vi "Configure PAS.vi"(8 "error in (no error)":errorcluster, 11 "Controller In":refnum<class "gController.lvclass">) -> ()   [LabVIEW 2017, in "Controller.lvlib" / "gController.lvclass"]
uses:
  gController.lvclass
  C:/Program Files (x86)/National Instruments/LabVIEW 2017/vi.lib/MSR Consulting, LLC/General Reuse/SuperActor/SuperActor.lvclass
  C:/Program Files (x86)/National Instruments/LabVIEW 2017/vi.lib/ActorFramework/Actor/Actor.lvclass
  Messages/Change Heater Ctl Params MSG/Change Heater Ctl Params.lvclass
  C:/Program Files (x86)/National Instruments/LabVIEW 2017/vi.lib/ActorFramework/Message/Message.lvclass
  Messages/Change Heater SP MSG/Change Heater SP MSG.lvclass
  Messages/Update PAS Enable Laser State/Update PAS Laser 0 Enable State MSG.lvclass
  G:/sw_repo/For Builds/Nicholas/Controller/Messages/Generic Boolean MSG/Generic Boolean Message.lvclass
  Messages/Enable PAS Laser 1 MSG/Update PAS Laser 1 Enable State MSG.lvclass
  PAS/Commands/Change Speaker State Cmd/Change Speaker State CMD.lvclass
  C:/Program Files (x86)/National Instruments/LabVIEW 2017/vi.lib/MSR Consulting, LLC/General Reuse/PAS/Commands/Change Speaker State CMD/Change Speaker State CMD.lvclass
  C:/Program Files (x86)/National Instruments/LabVIEW 2017/vi.lib/MSR Consulting, LLC/General Reuse/Command/Command.lvclass
  Messages/Forward Command/Forward Command MSG.lvclass
  <vilib>/MSR Consulting, LLC/General Reuse/Session APIs/File Access/Config Data/Config Data.lvclass
  <vilib>/MSR Consulting, LLC/General Reuse/PAS/Commands/Change Speaker State CMD/Change Speaker State CMD.lvclass/Change Speaker State CMD.ctl
  Messages/Forward Command/Forward Command MSG.lvclass/Forward Command MSG.ctl
  <vilib>/MSR Consulting, LLC/General Reuse/SuperActor/SuperActor.lvclass/SuperActor.ctl
  <vilib>/ActorFramework/Actor/Actor.lvclass/Actor.ctl
  <vilib>/ActorFramework/Message Enqueuer/Message Enqueuer.lvclass/Message Enqueuer.ctl
  <vilib>/MSR Consulting, LLC/General Reuse/Session APIs/File Access/Config Data/Config Data.lvclass/Config Data.ctl
  Messages/Change Heater Ctl Params MSG/Change Heater Ctl Params.lvclass/Change Heater Ctl Params.ctl
  Messages/Generic Boolean MSG/Generic Boolean Message.lvclass/Generic Boolean Message.ctl
  Messages/Change Heater SP MSG/Change Heater SP MSG.lvclass/Change Heater SP MSG.ctl
  <vilib>/MSR Consulting, LLC/General Reuse/SuperActor/Read Config Session.vi
  <vilib>/MSR Consulting, LLC/General Reuse/PAS/Commands/Change Speaker State CMD/Write cell.vi
  <vilib>/MSR Consulting, LLC/General Reuse/PAS/Commands/Change Speaker State CMD/Write state.vi
  Messages/Forward Command/Write CMD.vi
  Messages/Forward Command/Write id.vi
  <vilib>/MSR Consulting, LLC/General Reuse/Session APIs/File Access/Config Data/Accessors/Read Ref.vi
  Messages/Generic Boolean MSG/Write Bool.vi
  Messages/Change Heater SP MSG/Write id.vi
  Messages/Change Heater SP MSG/Write sp.vi
  Messages/Change Heater Ctl Params MSG/Write id.vi
  Messages/Change Heater Ctl Params MSG/Write ctl.vi
  <vilib>/ActorFramework/Message Enqueuer/Init from Existing Queue.vi
  <vilib>/MSR Consulting, LLC/General Reuse/Session APIs/File Access/Config Data/Read Array/Read DBL Array.vi
  <vilib>/MSR Consulting, LLC/General Reuse/Session APIs/File Access/Config Data/Read Array/Read Boolean Array.vi
  <vilib>/Utility/config.llb/Read Key (Double).vi
  <vilib>/ActorFramework/Message Priority Queue/Priority Enqueue.vi
  <vilib>/MSR Consulting, LLC/General Reuse/Session APIs/_Session Fwk/Session - Root.lvclass
  <vilib>/ActorFramework/Message Enqueuer/Message Enqueuer.lvclass
  <vilib>/Utility/config.llb/NI_LVConfig.lvlib
  <vilib>/ActorFramework/Actor/Actor.lvclass
panel:
  out "error out":errorcluster
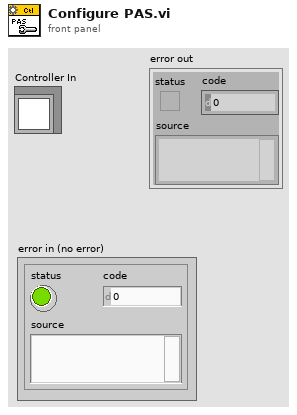
[diagram p1: front panel]
types:
  T1 = typedef "Session - Root.lvclass/Session Handle.ctl" = refnum<data-value>
  T2 = typedef "NI_LVConfig.lvlib/Config Data RefNum.ctl" = refnum<k1>
  T3 = cluster{"Read Array Data:DBL Data[0]":dbl, "Read Array Data:DBL Data[1]":dbl, "Read Array Data:DBL Data[2]":dbl}
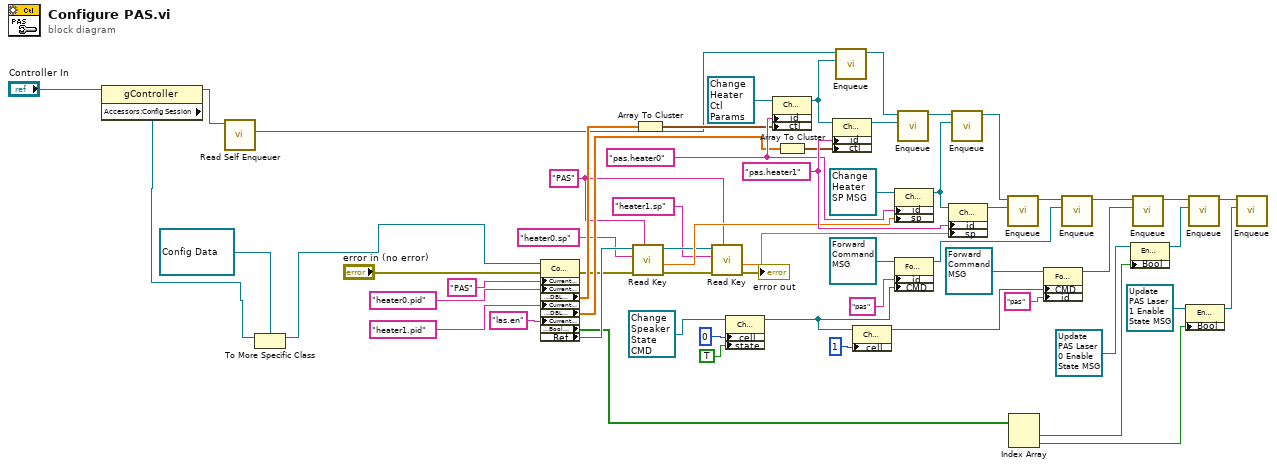
[diagram p0: block diagram]
diagram:
  w29 = "pas.heater1" ("id")
  w27 = "pas.heater0" ("id")
  w12 = "PAS" ("section")
  n1 = property class="gController"(reference="Controller In") -> (reference out=w2:refnum<class "gController.lvclass">, "Accessors:Config Session"=w5:T1)  [unwired: 1 in, 1 out]
  n2 = call <vilib>:"Read Self Enqueuer.vi"("Actor"=w2) -> ("Self Enqueuer"=w7:refnum<class "Message Enqueuer.lvclass">)  [unwired: 10 in]
  n3 = To More Specific Class(target class=refnum<data-value> refnum, reference=w5) -> (specific class reference=w4:refnum<data-value>)  [unwired: 1 in, 1 out]
  n4 = property class="Config Data"(reference=w4, error in="error in (no error)", "Current Section"="PAS", "Current Key"="heater0.pid", "Current Key"="heater1.pid", "Current Key"="las.en") -> (error out=w15:errorcluster, "Read Array Data:DBL Data"=w18:dbl[], "Read Array Data:DBL Data"=w22:dbl[], "Read Array Data:Bool Data"=w42:bool[], "Accessors:Ref"=w59:T2)  [unwired: 1 out]
  n5 = call-poly <vilib>:"Read Key.vi"("section"=w12, "error in (no error)"=w15, "key"="heater0.sp", "refnum"=w59) -> ("error out"=w16:errorcluster, "value"=w28:dbl, "refnum out"=w14:T2)  [unwired: 4 in, 1 out]
  n6 = Array To Cluster(array=w18) -> (cluster=w19:T3)
  n7 = call-poly <vilib>:"Read Key.vi"("section"=w12, "error in (no error)"=w16, "key"="heater1.sp", "refnum"=w14) -> ("error out"=→"error out":errorcluster, "value"=w30:dbl)  [unwired: 4 in, 2 out]
  n8 = property class="Change Speaker State CMD"(reference=refnum<class "Change Speaker State CMD.lvclass"> refnum ("gPAS Library.lvlib:Change Speaker State CMD"), "cell"=u8 0, "state"=TRUE) -> (reference out=w48:refnum<class "Change Speaker State CMD.lvclass">)  [unwired: 1 in, 1 out]
  n9 = property class="Change Heater Ctl Params"(reference=refnum<class "Change Heater Ctl Params.lvclass"> refnum ("Controller.lvlib:Change Heater Ctl Params"), "id"=w27, "ctl"=w19) -> (reference out=w21:refnum<class "Change Heater Ctl Params.lvclass">)  [unwired: 1 in, 1 out]
  n10 = Array To Cluster(array=w22) -> (cluster=w23:T3)
  n11 = property class="Change Heater Ctl Params"(reference=w21, "id"=w29, "ctl"=w23) -> (reference out=w24:refnum<class "Change Heater Ctl Params.lvclass">)  [unwired: 1 in, 1 out]
  n12 = call <vilib>:"Enqueue.vi"("Message"=w21, "Message Enqueuer in"=w7) -> ("Message Enqueuer out"=w20:refnum<class "Message Enqueuer.lvclass">)  [unwired: 8 in, 1 out]
  n13 = property class="Change Speaker State CMD"(reference=w48, "cell"=u8 1) -> (reference out=w50:refnum<class "Change Speaker State CMD.lvclass">)  [unwired: 1 in, 1 out]
  n14 = property class="Change Heater SP MSG"(reference=refnum<class "Change Heater SP MSG.lvclass"> refnum ("Controller.lvlib:Change Heater SP MSG"), "id"=w27, "sp"=w28) -> (reference out=w31:refnum<class "Change Heater SP MSG.lvclass">)  [unwired: 1 in, 1 out]
  n15 = property class="Forward Command MSG"(reference=refnum<class "Forward Command MSG.lvclass"> refnum ("Controller.lvlib:Forward Command MSG"), "id"="pas", "CMD"=w48) -> (reference out=w51:refnum<class "Forward Command MSG.lvclass">)  [unwired: 1 in, 1 out]
  n16 = call <vilib>:"Enqueue.vi"("Message"=w24, "Message Enqueuer in"=w20) -> ("Message Enqueuer out"=w58:refnum<class "Message Enqueuer.lvclass">)  [unwired: 8 in, 1 out]
  n17 = property class="Change Heater SP MSG"(reference=w31, "id"=w29, "sp"=w30) -> (reference out=w33:refnum<class "Change Heater SP MSG.lvclass">)  [unwired: 1 in, 1 out]
  n18 = call <vilib>:"Enqueue.vi"("Message"=w31, "Message Enqueuer in"=w58) -> ("Message Enqueuer out"=w32:refnum<class "Message Enqueuer.lvclass">)  [unwired: 8 in, 1 out]
  n19 = call <vilib>:"Enqueue.vi"("Message"=w33, "Message Enqueuer in"=w32) -> ("Message Enqueuer out"=w57:refnum<class "Message Enqueuer.lvclass">)  [unwired: 8 in, 1 out]
  n20 = Index Array(array=w42) -> (element #1=w35:bool, element #2=w37:bool)  [unwired: 2 in]
  n21 = property class="Forward Command MSG"(reference=refnum<class "Forward Command MSG.lvclass"> refnum ("Controller.lvlib:Forward Command MSG"), "CMD"=w50, "id"="pas") -> (reference out=w56:refnum<class "Forward Command MSG.lvclass">)  [unwired: 1 in, 1 out]
  n22 = call <vilib>:"Enqueue.vi"("Message"=w51, "Message Enqueuer in"=w57) -> ("Message Enqueuer out"=w54:refnum<class "Message Enqueuer.lvclass">)  [unwired: 8 in, 1 out]
  n23 = property class="Enable PAS Laser 0"(reference=refnum<class "Update PAS Laser 0 Enable State MSG.lvclass"> refnum ("Controller.lvlib:Enable PAS Laser 0"), "Bool"=w35) -> (reference out=w38:refnum<class "Update PAS Laser 0 Enable State MSG.lvclass">)  [unwired: 1 in, 1 out]
  n24 = call <vilib>:"Enqueue.vi"("Message"=w56, "Message Enqueuer in"=w54) -> ("Message Enqueuer out"=w55:refnum<class "Message Enqueuer.lvclass">)  [unwired: 8 in, 1 out]
  n25 = property class="Enable PAS Laser 1"(reference=refnum<class "Update PAS Laser 1 Enable State MSG.lvclass"> refnum ("Controller.lvlib:Enable PAS Laser 1"), "Bool"=w37) -> (reference out=w40:refnum<class "Update PAS Laser 1 Enable State MSG.lvclass">)  [unwired: 1 in, 1 out]
  n26 = call <vilib>:"Enqueue.vi"("Message"=w38, "Message Enqueuer in"=w55) -> ("Message Enqueuer out"=w39:refnum<class "Message Enqueuer.lvclass">)  [unwired: 8 in, 1 out]
  n27 = call <vilib>:"Enqueue.vi"("Message"=w40, "Message Enqueuer in"=w39) -> ()  [unwired: 8 in, 2 out]
